vi "set switch.vi"(8 "error in (no error)":errorcluster, 9 "state":bool, 10 "channel":dbl, 11 "SwitchBoxConrad in":refnum<class "SwitchBoxConrad.lvclass">) -> (0 "error out":errorcluster, 3 "SwitchBoxConrad out":refnum<class "SwitchBoxConrad.lvclass">)   [LabVIEW 2018, in "SwitchBoxConrad.lvclass"]
uses:
  SwitchBoxConrad.lvclass
  instrument.lvclass
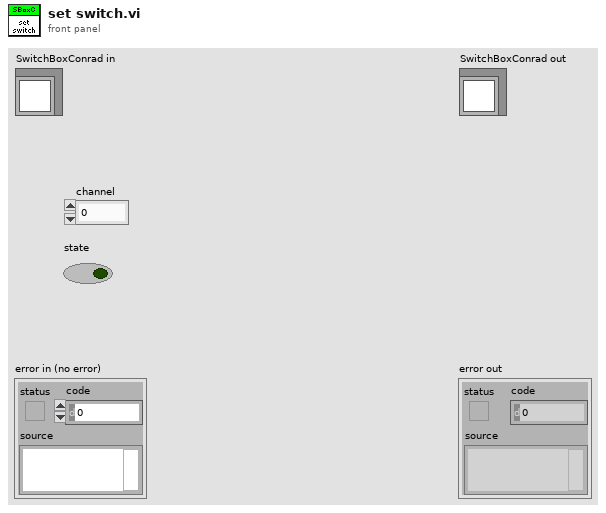
[diagram p1: front panel]
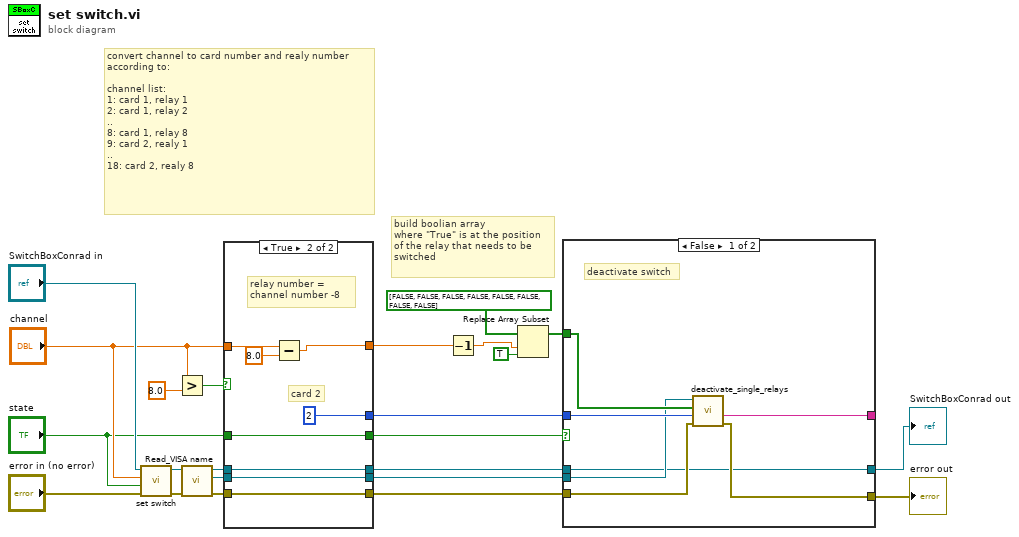
[diagram p0: block diagram]
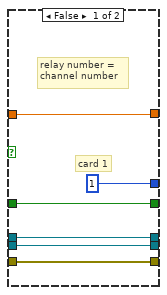
[diagram p2: hidden frame]
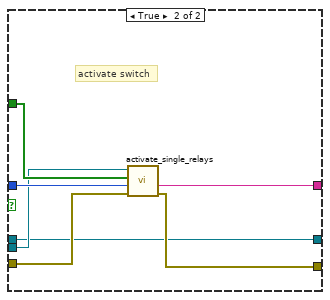
[diagram p3: hidden frame]
diagram:
  # "build boolian array\nwhere \"True\" is at the position\nof the relay that needs to be\nswitched"
  # "convert channel to card number and realy number\naccording to:\n\nchannel list:\n1: card 1, relay 1\n2: card 1, relay 2\n..\n8: card 1, relay 8\n9: card 2, realy 1\n..\n18: card 2, realy 8"
  n1 = call-parent "set switch.vi"("error in (no error)"="error in (no error)", "state"="state", "channel"="channel", "instrument in"="SwitchBoxConrad in") -> ("error out"=w12:errorcluster, "instrument out"=w13:refnum<class "SwitchBoxConrad.lvclass">)  [unwired: 6 in]
  n2 = Greater?(x="channel", y=8.0) -> (0:w20:bool)
  n3 = call-dynamic "Read_VISA name.vi"("error in (no error)"=w12, "instrument in"=w13) -> ("error out"=w10:errorcluster, "VISA resource name"=w9:refnum<visa-resource-name>, "instrument out"=w11:refnum<class "SwitchBoxConrad.lvclass">)  [unwired: 7 in]
  n4 = case shown="True" w20 {
    tunnel: "channel" -> [w24 w35]
    tunnel: w11 -> [w29 w37]
    tunnel: w10 -> [w28 w36]
    tunnel: [w29 w37] -> w18
    tunnel: [w28 w36] -> w17
    tunnel: [u8 1 u8 2] -> w16
    tunnel: "state" -> [w26 w32]
    tunnel: [w26 w32] -> w14
    tunnel: [w24 w30] -> w2
    tunnel: w9 -> [w25 w31]
    tunnel: [w25 w31] -> w8
    frame False {
      # "relay number =\nchannel number"
      # "card 1"
    }
    frame True {
      # "relay number =\nchannel number -8"
      # "card 2"
      n5 = Subtract(x=w35, y=8.0) -> (x-y=w30:dbl)
    }
  }
  n6 = Decrement(x=w2) -> (x-1=w1:dbl)
  n7 = Replace Array Subset(array=bool[] [FALSE, FALSE, FALSE, FALSE, FALSE, FALSE, FALSE, FALSE], new element=TRUE ("new element/subarray"), index=w1) -> (w5:bool[])
  n8 = case shown="False" w14 {
    tunnel: w17 -> [w41 w51]
    tunnel: w18 -> [w39 w46]
    tunnel: w16 -> [w44 w50]
    tunnel: w8 -> [w42 w48]
    tunnel: w5 -> [w43 w49]
    tunnel: [w40 w47] -> w4
    tunnel: [w39 w46] -> w3
    tunnel: [w38 w45] -> _
    frame False {
      # "deactivate switch"
      n9 = call "deactivate_single_relays.vi"("error in (no error)"=w41, "card address"=w44, "boolian array in"=w43, "VISA Refnum in"=w42) -> ("error out"=w40:errorcluster, "return string"=w38:string)  [unwired: 4 in, 2 out]
    }
    frame True {
      # "activate switch"
      n10 = call "activate_single_relays.vi"("error in (no error)"=w51, "card address"=w50, "boolian array in"=w49, "VISA Refnum in"=w48) -> ("error out"=w47:errorcluster, "return string"=w45:string)  [unwired: 4 in, 2 out]
    }
  }
  "error out" <- w4
  "SwitchBoxConrad out" <- w3
